vi "LCOS Queue Manager.vi"(0 "Queue":refnum<queue>, 2 "Queue States":cluster{"LCOS State":T2, "Data":variant}[](array[cluster]), 3 "error in (no error)":errorcluster, 4 "FNs":T1=enum."Front") -> (9 "error out":errorcluster)   [LabVIEW 2011]
uses:
  LCOS State Machine States.ctl
  LCOS Queue Management Actions.ctl
  LCOS Exit Global.vi
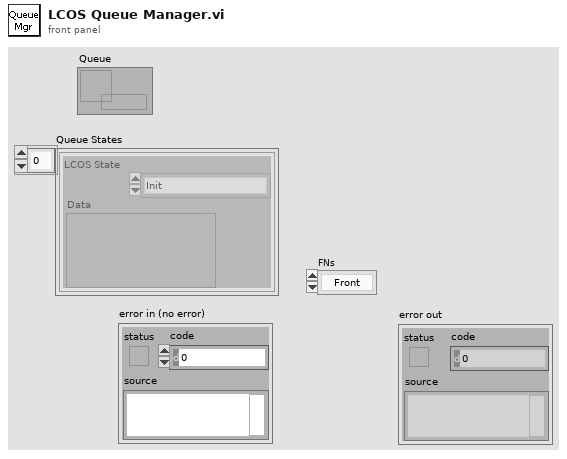
[diagram p1: front panel]
types:
  T1 = typedef "LCOS Queue Management Actions.ctl" = enum16{"Back", "Front", "Replace"}
  T2 = typedef "LCOS State Machine States.ctl" = enum16{"Init", "Idle", "Preview Button Pushed", "Update Button Pushed", "Pattern Selection Changed", "Pattern Definition Changed", "Selected File Changed", "Load Correction Pattern", "Load Correction Pattern Step 2", "Load User Pattern", "Load User Pattern Step 2", "Compute Pattern", "Correct Pattern", "Update Preview Display", "Update LCOS Display", "Error", "Clear Error", "Exit"}
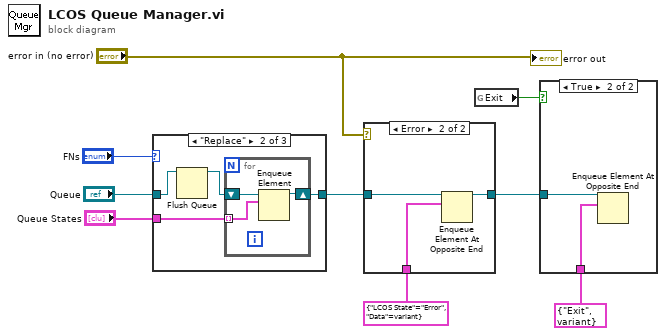
[diagram p0: block diagram]
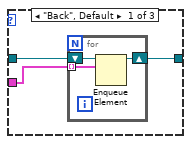
[diagram p4: hidden frame]
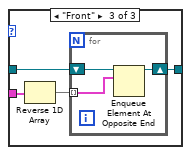
[diagram p5: hidden frame]
diagram:
  n1 = case shown="\"Replace\"" "FNs" {
    tunnel: "Queue" -> [w12 w19 w25]
    tunnel: "Queue States" -> [w11 w16 w26]
    tunnel: [w10 w17 w24] -> w5
    frame "Back", Default {
      n2 = for {
        tunnel: w11 -> [w14] mode=indexing
        shift-right: [w13] -> w10
        shift-left: w12 -> [w15]
        n3 = Enqueue Element(queue=w15, element=w14) -> (queue out=w13:refnum<queue>)  [unwired: 2 in, 2 out]
      }
    }
    frame "Replace" {
      n4 = Flush Queue(queue=w19) -> (queue out=w18:refnum<queue>)  [unwired: 1 in, 2 out]
      n5 = for {
        shift-right: [w21] -> w17
        shift-left: w18 -> [w22]
        tunnel: w16 -> [w20] mode=indexing
        n6 = Enqueue Element(queue=w22, element=w20) -> (queue out=w21:refnum<queue>)  [unwired: 2 in, 2 out]
      }
    }
    frame "Front" {
      n7 = Reverse 1D Array(array=w26) -> (reversed array=w23:cluster{"LCOS State":T2, "Data":variant}[])
      n8 = for {
        shift-right: [w28] -> w24
        shift-left: w25 -> [w29]
        tunnel: w23 -> [w27] mode=indexing
        n9 = Enqueue Element At Opposite End(queue=w29, element=w27) -> (queue out=w28:refnum<queue>)  [unwired: 2 in, 2 out]
      }
    }
  }
  n10 = case shown="Error" "error in (no error)" {
    tunnel: w5 -> [w30 w33]
    tunnel: [w30 w32] -> w3
    tunnel: cluster{"LCOS State":T2, "Data":variant} {"LCOS State"=enum."Error", "Data"=variant} ("element") -> [_ w31]
    frame No Error {
    }
    frame Error {
      n11 = Enqueue Element At Opposite End(queue=w33, element=w31) -> (queue out=w32:refnum<queue>)  [unwired: 2 in, 2 out]
    }
  }
  n12 = global read "LCOS Exit Global.vi" "Exit"() -> (w4:bool)
  n13 = case shown="True" w4 {
    tunnel: w3 -> [_ w35]
    tunnel: cluster{"LCOS State":T2, "Data":variant} {"LCOS State"=enum."Exit", "Data"=variant} ("element") -> [_ w34]
    frame False {
    }
    frame True {
      n14 = Enqueue Element At Opposite End(queue=w35, element=w34) -> ()  [unwired: 2 in, 3 out]
    }
  }
  "error out" <- "error in (no error)"
